vi "Set ErrorQ on Variant.vi"(8 "error in (no error)":errorcluster, 10 "Queue in":T1, 11 "Variant in":variant) -> (0 "error out":errorcluster, 2 "replaced":bool, 3 "Variant out":variant)   [LabVIEW 2020, in "Internal Comm Classes.lvlib" / "WPL Comm.lvclass"]
uses:
  WPL Comm.lvclass
  Waveform error queue.ctl
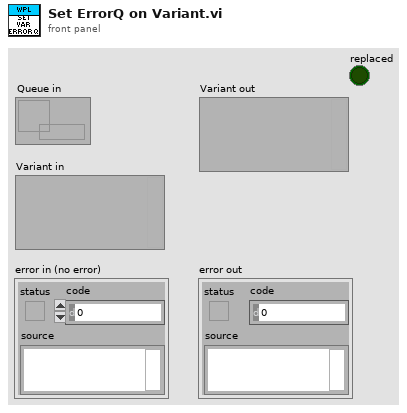
[diagram p1: front panel]
types:
  T1 = typedef "Internal Comm Classes.lvlib/WPL Comm.lvclass/Waveform error queue.ctl" = refnum<queue>
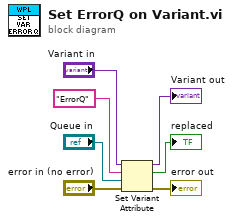
[diagram p0: block diagram]
diagram:
  n1 = Set Variant Attribute(Variant="Variant in", name="ErrorQ", value="Queue in", error in="error in (no error)") -> (Variant out=→"Variant out":variant, replaced=→"replaced":bool, error out=→"error out":errorcluster)
